vi "test3-1ToNBroadcastStatus.vi"(8 "error in (no error)":errorcluster, 11 "TestCase in":refnum<class "testcase-CSMBroadcast.lvclass">) -> (0 "error out":errorcluster, 3 "TestCase out":refnum<class "testcase-CSMBroadcast.lvclass">)   [LabVIEW 2017, in "testcase-CSMBroadcast.lvclass"]
uses:
  testcase-CSMBroadcast.lvclass
  0b17d103-e67b-41be-a9eb-a2ee1311ff1f.vi
  5999693e-4f8a-4b34-ae87-f34dff5771be.vi
  src/user.lib/_NEVSTOP/Communicable State Machine(CSM)/AdvanceAPI/CSM - Get Module Attribute.vi
  <vilib>/addons/_JKI Toolkits/VI Tester/TestCase.llb/TestCase.lvclass
  src/user.lib/_NEVSTOP/Communicable State Machine(CSM)/Communicable State Machine.lvlib
  C:/Program Files (x86)/National Instruments/LabVIEW 2017/vi.lib/addons/_JKI Toolkits/VI Tester/TestCase.llb/TestCase.lvclass
panel:
  out "LoopCount2":i32
  out "LoopCount":i32
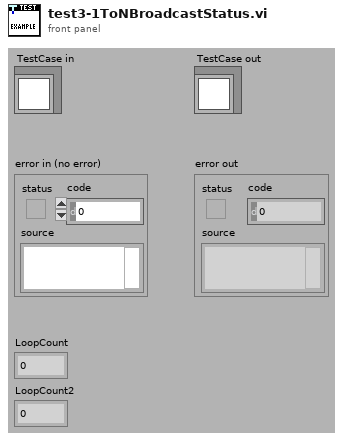
[diagram p1: front panel]
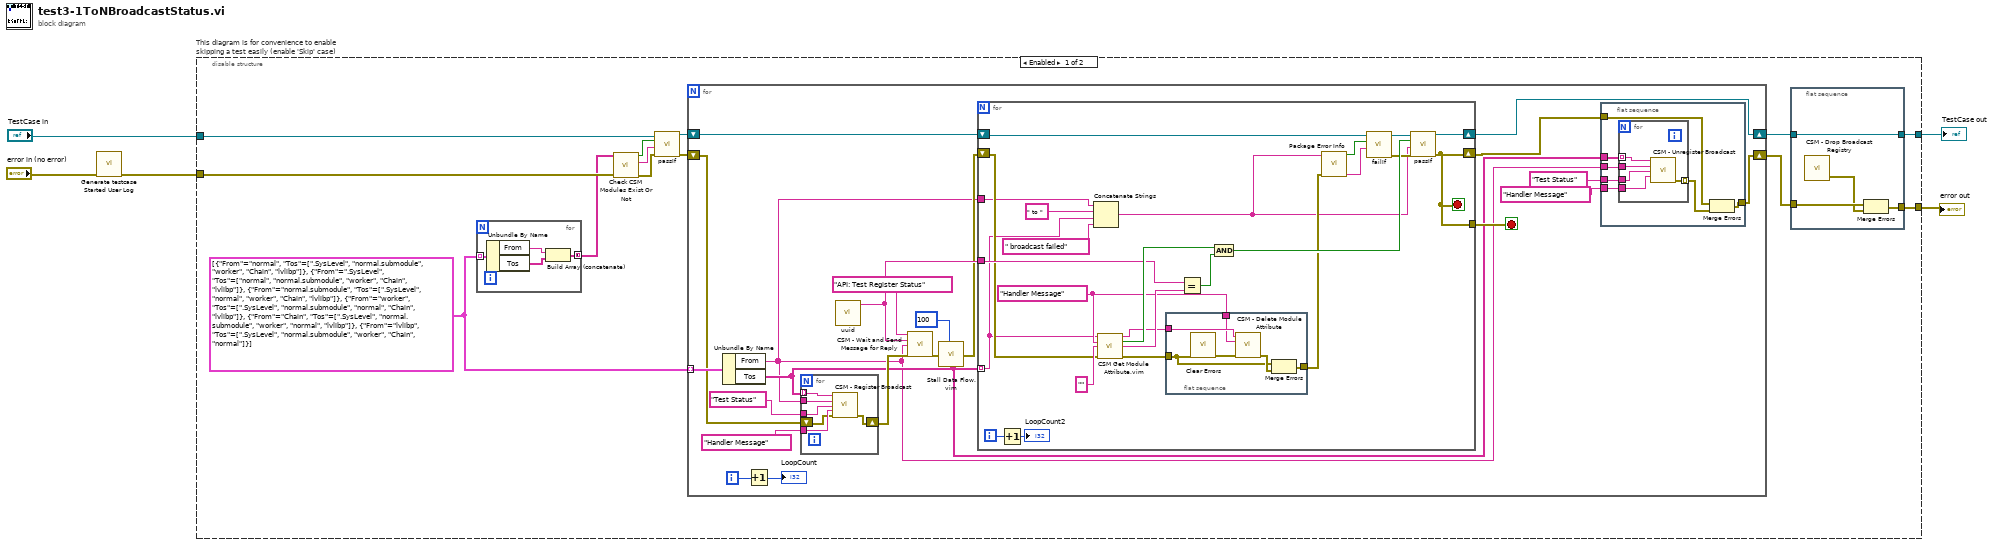
[diagram p0: block diagram]
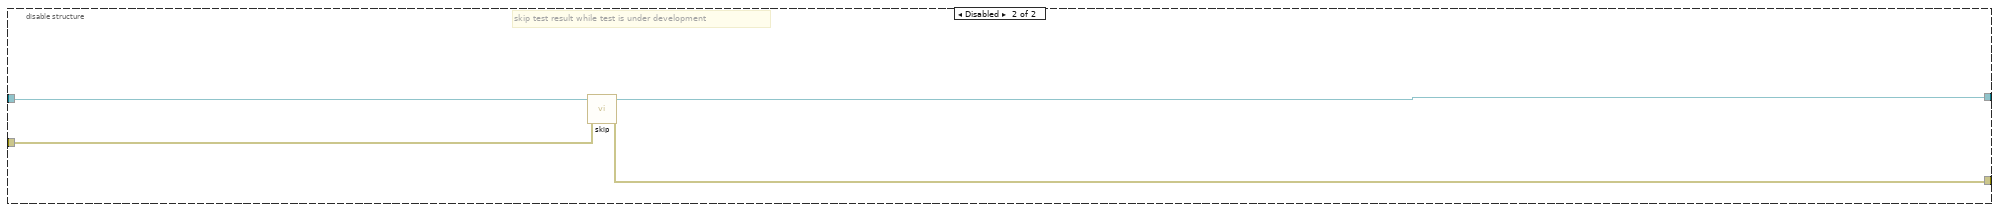
[diagram p2: hidden frame]
diagram:
  n1 = call "Generate testcase Started User Log.vi"("Error In"="error in (no error)") -> ("error out"=w1:errorcluster)  [unwired: 10 in]
  n2 = disable-structure "This diagram is for convenience to enable skipping a test easily (enable 'Skip' case)" shown="Enabled" {
    disable-tunnel: "TestCase in" -> [w11 w100]
    disable-tunnel: [w6 w98] -> w2
    disable-tunnel: [w17 w99] -> w4
    disable-tunnel: w1 -> [w13 w97]
    frame Enabled {
      w9 = cluster{"From":string, "Tos":string[]}[] [{"From"="normal", "Tos"=[".SysLevel", "normal.submodule", "worker", "Chain", "lvlibp"]}, {"From"=".SysLevel", "Tos"=["normal", "normal.submodule", "worker", "Chain", "lvlibp"]}, {"From"="normal.submodule", "Tos"=[".SysLevel", "normal", "worker", "Chain", "lvlibp"]}, {"From"="worker", "Tos"=[".SysLevel", "normal.submodule", "normal", "Chain", "lvlibp"]}, {"From"="Chain", "Tos"=[".SysLevel", "normal.submodule", "worker", "normal", "lvlibp"]}, {"From"="lvlibp", "Tos"=[".SysLevel", "normal.submodule", "worker", "Chain", "normal"]}]
      n3 = for {
        tunnel: w9 -> [w22] mode=indexing
        tunnel: [w19] -> w8 mode=concatenating
        n4 = Unbundle By Name(w22) -> ("From"=w21:string, "Tos"=w20:string[])
        n5 = Build Array (concatenate)(w21, w20) -> (w19:string[])
      }
      n6 = call "Check CSM Modules Exist Or Not.vi"("error in"=w13, "CSM names in"=w8) -> ("error out"=w14:errorcluster, "Debug string"=w15:string, "All Modules Exist?"=w16:bool)  [unwired: 7 in]
      n7 = call-dynamic "passIf.vi"("error in (no error)"=w14, "message (\"\")"=w15, "pass"=w16, "TestCase in"=w11) -> ("error out"=w12:errorcluster, "TestCase out"=w10:refnum<class "testcase-CSMBroadcast.lvclass">)  [unwired: 6 in]
      n8 = for {
        shift-right: [w35] -> w18
        shift-left: w12 -> [w30]
        shift-right: [w31] -> w7
        shift-left: w10 -> [w40]
        tunnel: w9 -> [w45] mode=indexing
        i -> [w47]
        stop <- w39 stop-if-true
        n9 = Unbundle By Name(w45) -> ("From"=w27:string, "Tos"=w34:string[])
        n10 = Increment(x=w47) -> (x+1=→"LoopCount":i32)
        n11 = for {
          tunnel: w27 -> [w96]
          tunnel: w34 -> [w95] mode=indexing
          tunnel: "Test Status" -> [w94]
          tunnel: "Handler Message" -> [w93]
          shift-right: [w92] -> w36
          shift-left: w30 -> [w91]
          n12 = call "CSM - Register Broadcast.vi"("CSM Name(Empty for Broadcast Event)"=w95, "Source CSM Name (* as Default)"=w96, "Trigger"=w94, "API (If \"\", Same as Trigger)"=w93, "Error In"=w91) -> ("error out"=w92:errorcluster)  [unwired: 9 in, 1 out]
        }
        n13 = call "uuid.vi"() -> ("UUID"=w41:string)  [unwired: 11 in]
        n14 = call "CSM - Wait and Send Message for Reply.vi"("State"="API: Test Register Status", "Arguments (\"\")"=w41, "Target Module"=w27, "Error In (No Error)"=w36) -> ("error out"=w43:errorcluster)  [unwired: 8 in, 3 out]
        n15 = call "Stall Data Flow.vim"("value in"=w43, "milliseconds to wait"=u32 100) -> ("value out"=w29:errorcluster)  [unwired: 1 out]
        n16 = for {
          tunnel: w41 -> [w82]
          tunnel: [w71] -> w39
          shift-right: [w80] -> w31
          shift-left: w40 -> [w64]
          shift-right: [w71] -> w28
          shift-left: w29 -> [w72]
          tunnel: w34 -> [w69] mode=indexing
          tunnel: w27 -> [w68]
          i -> [w74]
          stop <- w71 stop-if-true
          w75 = "Handler Message" ("To")
          n17 = Increment(x=w74) -> (x+1=→"LoopCount2":i32)
          n18 = Concatenate Strings(w68, " to " ("string"), w69, " broadcast failed" ("string")) -> (w60:string)
          n19 = call "CSM Get Module Attribute.vim"("CSM Name"=w69, "Attribute"=w75, "Default Value (Empty Variant)"="", "Error In"=w72) -> ("CSM Name (Dup)"=w76:string, "Found"=w84:bool, "Value"=w81:string, "error out"=w77:errorcluster)  [unwired: 7 in, 1 out]
          n20 = flat-sequence {
            tunnel: w77 -> [w86]
            tunnel: w76 -> [w89]
            tunnel: w75 -> [w88]
            tunnel: [w85] -> w61
            frame #0 {
              n21 = call <vilib>:"Clear Errors.vi"("error in (no error)"=w86) -> ("error out"=w90:errorcluster)  [unwired: 5 in, 1 out]
              n22 = call "CSM - Delete Module Attribute.vi"("CSM Name"=w89, "Attribute"=w88, "Error In"=w90) -> ("error out"=w87:errorcluster)  [unwired: 9 in, 3 out]
              n23 = Merge Errors(w86, w87) -> (w85:errorcluster)
            }
          }
          n24 = Equal?(x=w82, y=w81) -> (x = y?=w79:bool)
          n25 = And(x=w84, y=w79) -> (x .and. y?=w78:bool)
          n26 = call "Package Error Info.vi"("error in"=w61, "String in"=w60) -> ("packed error info out"=w65:string, "error status"=w66:bool)  [unwired: 8 in]
          n27 = call-dynamic "failIf.vi"("message (\"\")"=w65, "fail"=w66, "TestCase in"=w64) -> ("error out"=w62:errorcluster, "TestCase out"=w63:refnum<class "testcase-CSMBroadcast.lvclass">)  [unwired: 7 in]
          n28 = call-dynamic "passIf.vi"("error in (no error)"=w62, "message (\"\")"=w60, "pass"=w78, "TestCase in"=w63) -> ("error out"=w71:errorcluster, "TestCase out"=w80:refnum<class "testcase-CSMBroadcast.lvclass">)  [unwired: 6 in]
        }
        n29 = flat-sequence {
          tunnel: [w54] -> w35
          tunnel: w34 -> [w53]
          tunnel: w27 -> [w52]
          tunnel: "Test Status" -> [w51]
          tunnel: "Handler Message" -> [w49]
          tunnel: w28 -> [w48]
          frame #0 {
            n30 = for {
              tunnel: w53 -> [w59] mode=indexing
              tunnel: w52 -> [w58]
              tunnel: w51 -> [w57]
              tunnel: [w56] -> w50 mode=indexing
              tunnel: w49 -> [w55]
              n31 = call "CSM - Unregister Broadcast.vi"("CSM Name(Empty for Broadcast Event)"=w59, "Source CSM Name (* as Default)"=w58, "Trigger"=w57, "API (\"*\" as Default)"=w55) -> ("error out"=w56:errorcluster)  [unwired: 10 in, 1 out]
            }
            n32 = Merge Errors(w48, w50) -> (w54:errorcluster)
          }
        }
      }
      n33 = flat-sequence {
        tunnel: [w26] -> w17
        tunnel: w18 -> [w25]
        tunnel: [w23] -> w6
        tunnel: w7 -> [w23]
        frame #0 {
          n34 = call "CSM - Drop Broadcast Registry.vi"() -> ("error out"=w24:errorcluster)  [unwired: 15 in]
          n35 = Merge Errors(w25, w24) -> (w26:errorcluster)
        }
      }
    }
    frame Disabled {
      # "skip test result while test is under development"
      n36 = call <vilib>:"skip.vi"("error in (no error)"=w97, "TestCase in"=w100) -> ("error out"=w99:errorcluster, "TestCase out"=w98:refnum<class "testcase-CSMBroadcast.lvclass">)  [unwired: 8 in]
    }
  }
  "error out" <- w4
  "TestCase out" <- w2
